vi "Get run time chain.vi"(8 "error in (no error)":errorcluster, 11 "Cascade512II Basein":refnum<class "DAQCascade512II.lvclass">) -> (0 "error out":errorcluster, 2 "run time":variant[](array[variant]), 3 "Cascade512II Baseout":refnum<class "DAQCascade512II.lvclass">)   [LabVIEW 2012, in "DAQCascade512II.lvclass"]
uses:
  DAQCascade512II.lvclass
  DAQCascade512II.lvclass/DAQCascade512II.ctl
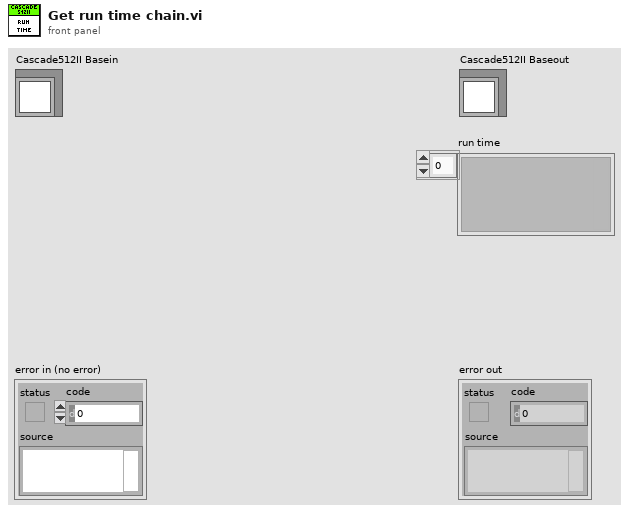
[diagram p1: front panel]
types:
  T1 = typedef "DAQCascade512II.lvclass/run_time cluster.ctl" = cluster{"Camera Handle":u32, "Y dimension":u32, "X dimension":u32, "Image Handle":u32, "Display Handle":u32, "File Handle":u32, "saved frames":dbl, "intialized?":bool, "continue_acquiring?":bool, "Image":T2, "image queue":refnum<queue>, "TTL iteration":i32, "get images from queue reference":refnum<vi>, "get image vi ref":refnum<vi>}
  T2 = typedef "IMAQ Image.ctl" = refnum<image>
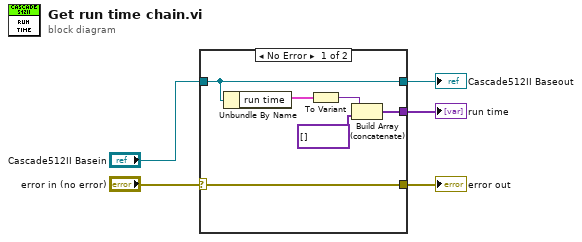
[diagram p0: block diagram]
diagram:
  n1 = case shown="No Error" "error in (no error)" {
    selector: "error in (no error)" -> [w6 w12]
    tunnel: [w11 _] -> w3
    tunnel: "Cascade512II Basein" -> [w10 w13]
    tunnel: [w10 w13] -> w4
    tunnel: [w6 w12] -> w5
    frame No Error {
      n2 = Unbundle By Name(w10) -> ("run time"=w9:T1)
      n3 = To Variant(anything=w9) -> (Variant=w8:variant)
      n4 = Build Array (concatenate)(w8, variant[] [] ("array")) -> (w11:variant[])
    }
    frame Error {
    }
  }
  "error out" <- w5
  "Cascade512II Baseout" <- w4
  "run time" <- w3
